vi "Gradient.vi"(7 "Percent":dbl=1.0, 10 "End Color":u32(colorbox)=16777238, 11 "Start Color":u32(colorbox)) -> (3 "Gradient Color":u32(colorbox))   [LabVIEW 2015, in "StatusHistory.lvclass"]
doc: "<b> </b> <b> </b>\n©2016 Q Software Innovations, LLC (QSI)\nwritten by Quentin Alldredge\nproduced in LabVIEW 2015\n\nsupport@qsoftwareinnovations.com\nwww.qsoftwareinnovations.com\n\nAll rights reserved.\n\nRedistribution and use in source and binary forms, with or without modification, are permitted provided that the following conditions are met:\n\n * Redistributions of source code must retain the above copyright notice, this list of conditions and the following disclaimer.\n * Redistributions in binary form must reproduce the above copyright notice, this list of conditions and the following disclaimer in the documentation and/or other materials provided with the distribution.\n * Neither the name of Q Software Innovations, LLC. nor the names of its contributors may be used to endorse or promote products derived from this software without specific prior written permission.\n\nTHIS SOFTWARE IS PROVIDED BY THE COPYRIGHT HOLDERS AND CONTRIBUTORS \"AS IS\" AND ANY EXPRESS OR IMPLIED WARRANTIES, INCLUDING, BUT NOT LIMITED TO, THE IMPLIED WARRANTIES OF MERCHANTABILITY AND FITNESS FOR A PARTICULAR PURPOSE ARE DISCLAIMED. IN NO EVENT SHALL THE COPYRIGHT OWNER OR CONTRIBUTORS BE LIABLE FOR ANY DIRECT, INDIRECT, INCIDENTAL, SPECIAL, EXEMPLARY, OR CONSEQUENTIAL DAMAGES (INCLUDING, BUT NOT LIMITED TO, PROCUREMENT OF SUBSTITUTE GOODS OR SERVICES; LOSS OF USE, DATA, OR PROFITS; OR BUSINESS INTERRUPTION) HOWEVER CAUSED AND ON ANY THEORY OF LIABILITY, WHETHER IN CONTRACT, STRICT LIABILITY, OR TORT (INCLUDING NEGLIGENCE OR OTHERWISE) ARISING IN ANY WAY OUT OF THE USE OF THIS SOFTWARE, EVEN IF ADVISED OF THE POSSIBILITY OF SUCH DAMAGE."
uses:
  StatusHistory.lvclass
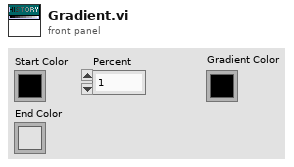
[diagram p1: front panel]
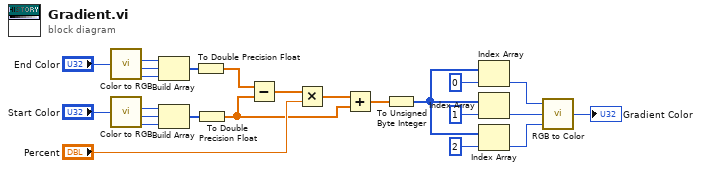
[diagram p0: block diagram]
diagram:
  n1 = call <vilib>:"Color to RGB.vi"("Color"="End Color") -> ("R"=w22:u8, "G"=w21:u8, "B"=w20:u8)  [unwired: 1 out]
  n2 = call <vilib>:"Color to RGB.vi"("Color"="Start Color") -> ("R"=w19:u8, "G"=w18:u8, "B"=w17:u8)  [unwired: 1 out]
  n3 = Build Array(w22, w21, w20) -> (w16:u8[])
  n4 = Build Array(w19, w18, w17) -> (w15:u8[])
  n5 = To Double Precision Float(number=w16) -> (double precision float=w13:dbl[])
  n6 = To Double Precision Float(number=w15) -> (double precision float=w3:dbl[])
  n7 = Subtract(x=w13, y=w3) -> (x-y=w4:dbl[])
  n8 = Multiply(x=w4, y="Percent") -> (x*y=w2:dbl[])
  n9 = Add(x=w2, y=w3) -> (x+y=w1:dbl[])
  n10 = To Unsigned Byte Integer(number=w1) -> (unsigned 8bit integer=w7:u8[])
  n11 = Index Array(array=w7, index=0) -> (element=w12:u8)
  n12 = Index Array(array=w7, index=1) -> (element=w11:u8)
  n13 = Index Array(array=w7, index=2) -> (element=w10:u8)
  n14 = call <vilib>:"RGB to Color.vi"("B"=w10, "G"=w11, "R"=w12) -> ("Color"=→"Gradient Color":u32)
